vi "can_stopDaemon.vi"(8 "error in (no error)":errorcluster, 11 "Instrument in":refnum<class "Instrument.lvclass">) -> (0 "error out":errorcluster, 3 "Instrument out":refnum<class "Instrument.lvclass">)   [LabVIEW 2019, in "Instrument.lvclass"]
uses:
  Instrument.lvclass
  Instrument.lvclass/Instrument.ctl
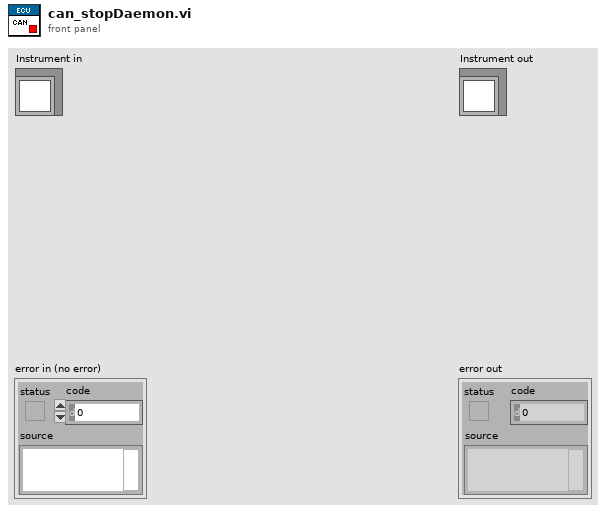
[diagram p1: front panel]
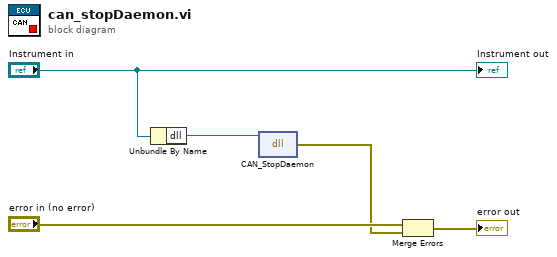
[diagram p0: block diagram]
diagram:
  n1 = Unbundle By Name("Instrument in") -> ("dll"=w2:path)
  n2 = dll-call lib="C:/Dev/22KW-Dyno/software/data/DynoAPI.dll" fn="CAN_StopDaemon"(path in=w2) -> (error out=w1:errorcluster)  [unwired: 3 in, 1 out]
  n3 = Merge Errors("error in (no error)", w1) -> (→"error out":errorcluster)
  "Instrument out" <- "Instrument in"
